vi "Close.vi"(8 "error in (no error)":errorcluster, 11 "AirCondition in":refnum<class "AirCondition.lvclass">) -> (0 "error out":errorcluster, 3 "AirCondition out":refnum<class "AirCondition.lvclass">)   [LabVIEW 2013, in "AirCondition.lvclass"]
uses:
  AirCondition.lvclass
  AirCondition.lvclass/AirCondition.ctl
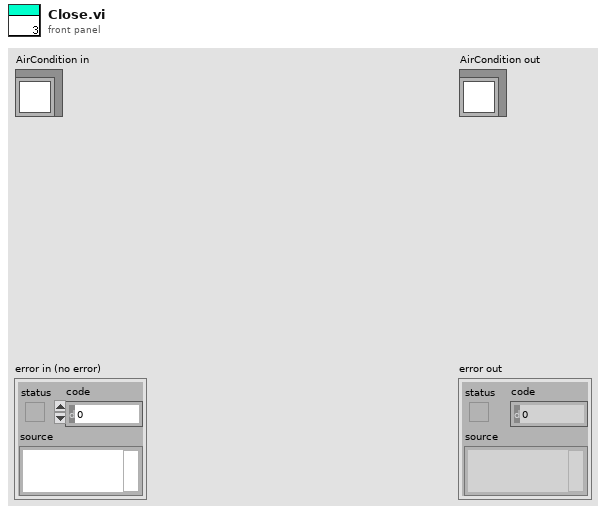
[diagram p1: front panel]
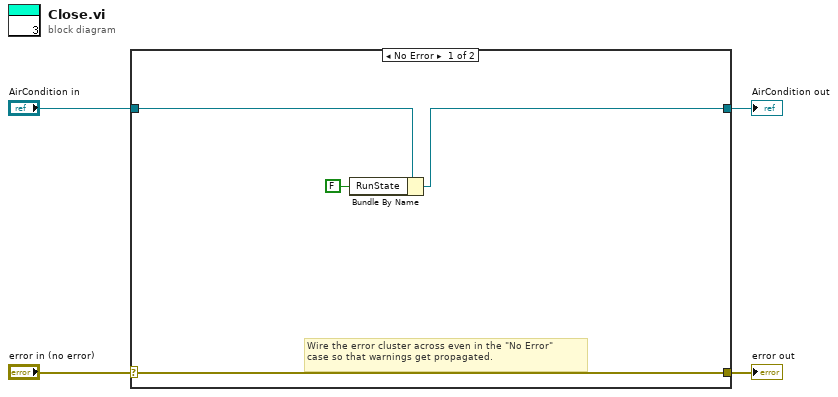
[diagram p0: block diagram]
diagram:
  n1 = case shown="No Error" "error in (no error)" {
    selector: "error in (no error)" -> [w8 w10]
    tunnel: [w8 w10] -> w3
    tunnel: [w5 w9] -> w1
    tunnel: "AirCondition in" -> [w6 w9]
    frame No Error {
      # "Wire the error cluster across even in the \"No Error\"\ncase so that warnings get propagated."
      n2 = Bundle By Name(cluster=w6, "RunState"=FALSE) -> (w5:refnum<class "AirCondition.lvclass">)
    }
    frame Error {
    }
  }
  "error out" <- w3
  "AirCondition out" <- w1
